vi "CameraTesting3.vi"() -> ()   [LabVIEW 2019]
doc: "The myRIO Project template acquires acceleration data from the onboard accelerometer and displays the changes of acceleration values in a waveform chart."
uses:
  <vilib>/myRIO/Express VI/Onboard IO/Encoder/Encoder Express VI.xnode
  <vilib>/myRIO/Common/Instrument Driver Framework/myRIO v1.0/Encoder/typedefs/Encoder Count Direction Enum.ctl
  <vilib>/myRIO/Instrument Drivers/Onboard IO/Encoder/typedefs/Encoder Reference.ctl
  <vilib>/myRIO/Instrument Drivers/Onboard IO/Encoder/Encoder.lvlib
  <vilib>/myRIO/Common/Instrument Driver Framework/myRIO v1.0/Encoder/typedefs/Encoder Channels Enum.ctl
  <vilib>/myRIO/Common/Instrument Driver Framework/Utilities/typedefs/myRIO Generic Hardware Reference.ctl
  <vilib>/myRIO/Common/Instrument Driver Framework/Utilities/typedefs/myRIO v1.0 Reference.ctl
  <vilib>/myRIO/Common/Instrument Driver Framework/Utilities/typedefs/Generic FPGA Reference.ctl
  <vilib>/myRIO/Common/Instrument Driver Framework/Utilities/typedefs/Hardware Version Enum.ctl
  <vilib>/myRIO/Common/Instrument Driver Framework/myRIO v1.0/Encoder/typedefs/Encoder Signal Mode.ctl
  <vilib>/myRIO/Instrument Drivers/Onboard IO/Encoder/vis/Read.vi
  <vilib>/myRIO/Instrument Drivers/Onboard IO/Encoder/vis/myRIO Encoder Open.xnode
  <vilib>/userdefined/High Color/nirio_resource_hc.ctl
  <vilib>/myRIO/Common/Instrument Driver Framework/myRIO v1.0/Encoder/typedefs/Encoder Configuration v1.0.ctl
  <vilib>/myRIO/Common/Instrument Driver Framework/myRIO v1.0/Encoder/vis/myRIO v1.1 Open Encoder.vi
  <vilib>/myRIO/Common/Instrument Driver Framework/myRIO v1.0/Encoder/vis/myRIO v1.0 Configure Encoder.vi
  <vilib>/myRIO/Common/Instrument Driver Framework/Utilities/vis/Is FPGA Ref Available.vi
  <vilib>/myRIO/Express VI/Onboard IO/DO/DO Express VI.xnode
  <vilib>/myRIO/Instrument Drivers/Onboard IO/DIO/typedefs/DIO Reference.ctl
  <vilib>/myRIO/Instrument Drivers/Onboard IO/DIO/DIO.lvlib
  <vilib>/myRIO/Common/Instrument Driver Framework/myRIO v1.0/DIO/typedefs/DIO Channels List.ctl
  <vilib>/myRIO/Common/Instrument Driver Framework/myRIO v1.0/DIO/typedefs/DIO Channels Enum.ctl
  <vilib>/myRIO/Instrument Drivers/Onboard IO/DIO/vis/Write.vi
  <vilib>/myRIO/Instrument Drivers/Onboard IO/DIO/vis/myRIO DIO Open.xnode
  <vilib>/myRIO/Common/Instrument Driver Framework/myRIO v1.0/DIO/vis/myRIO v1.1 Open DIO.vi
  <vilib>/Analysis/NI_AALBase.lvlib
panel:
  out "Pause":i32
  out "WaitTime":dbl=1000.0
  out "SquareWave":dbl
  out "FrameRate":i32=30
  out "Stop":bool
  out "VidTS":dbl[][](array[numeric])
  out "GoVid":i32=1
  out "VidFrameClock":i32
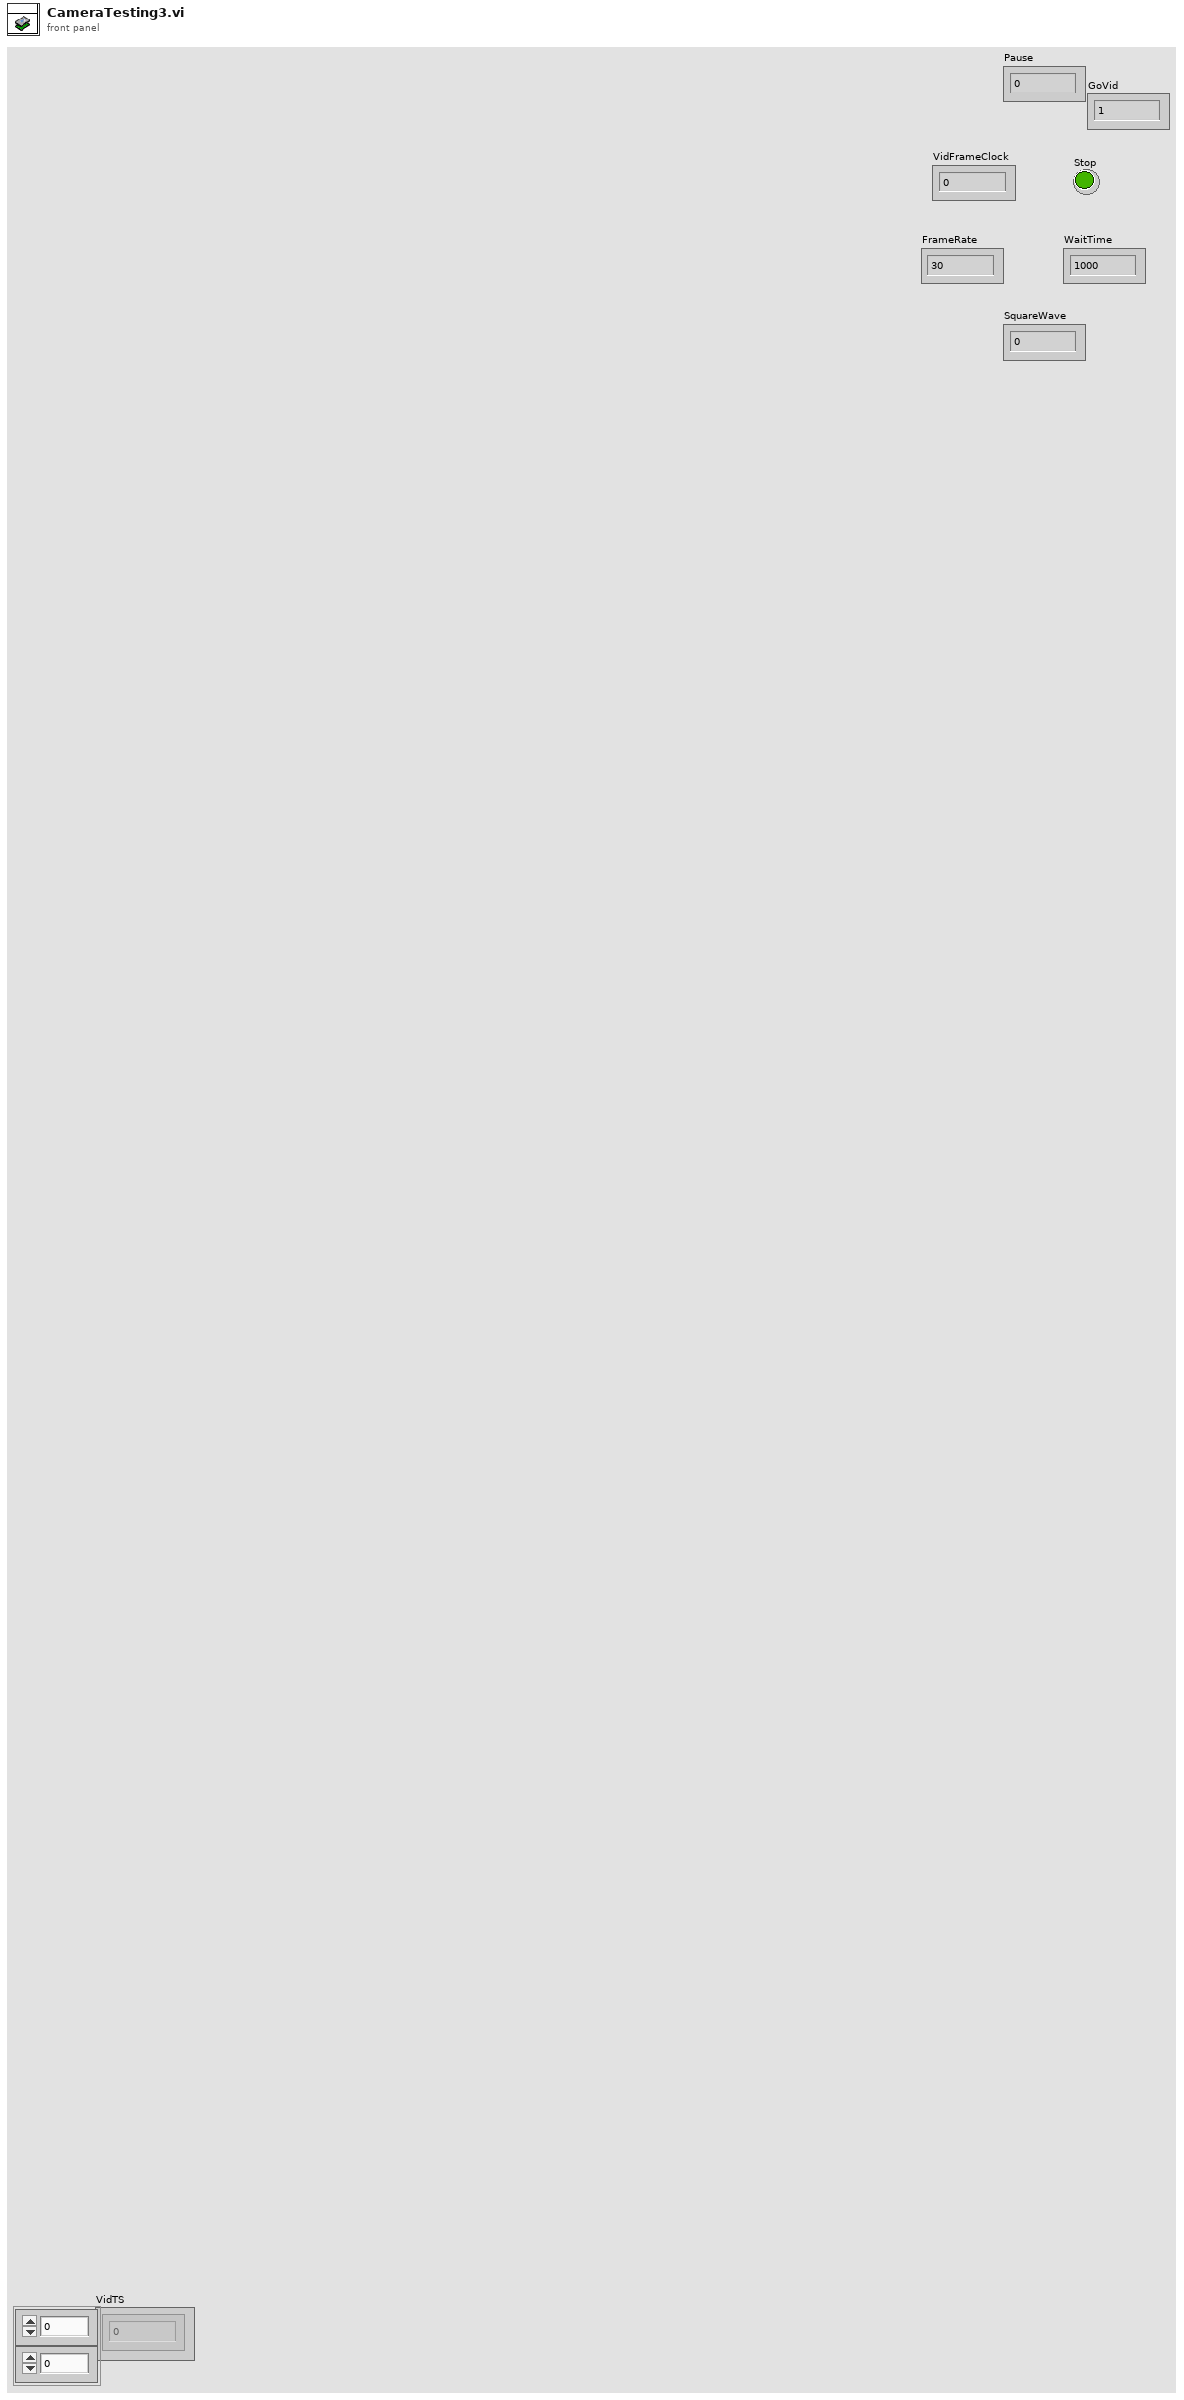
[diagram p1: front panel]
types:
  T1 = typedef "Encoder.lvlib/Encoder Reference.ctl" = cluster{"myRIO Reference":T2, "Encoder Channels Enum":T6}
  T2 = typedef "myRIO Generic Hardware Reference.ctl" = cluster{"myRIO Model":T3, "myRIO Hardware Reference":T4}
  T3 = typedef "Hardware Version Enum.ctl" = enum16{"Unknown", "myRIO-1900", "myRIO-1950", "roboRIO", "NI ELVIS RIO CM", "ELVIS III"}
  T4 = typedef "myRIO v1.0 Reference.ctl" = cluster{"Generic FPGA Reference":T5, "Allow multiple opens":bool}
  T5 = typedef "Generic FPGA Reference.ctl" = refnum<k20>
  T6 = typedef "Encoder Channels Enum.ctl" = enum16{"Not Connected", "C/ENC0", "C/ENC1", "A/ENC", "A/ENC0", "A/ENC1", "A/ENC2", "A/ENC3", "A/ENC4", "A/ENC5", "A/ENC6", "A/ENC7", "A/ENC8", "A/ENC9", "B/ENC", "B/ENC0", "B/ENC1", "B/ENC2", "B/ENC3", "B/ENC4", "B/ENC5", "B/ENC6", "B/ENC7", "B/ENC8", "B/ENC9", "DIO/ENC0", "DIO/ENC1", "DIO/ENC2", "DIO/ENC3", "DIO/ENC4"}
  T7 = typedef "Encoder Signal Mode.ctl" = enum16{"Quadrature phase signal", "Step and direction signal"}
  T8 = typedef "nirio_resource_hc.ctl" = tag
  T9 = typedef "NI_Matrix.lvlib/RealMatrix.ctl" = dbl[][]
  T10 = typedef "DIO.lvlib/DIO Reference.ctl" = cluster{"myRIO Reference":T2, "DIO Channels List":T11}
  T11 = typedef "DIO Channels List.ctl" = T12[]
  T12 = typedef "DIO Channels Enum.ctl" = enum16{"Not Connected", "C/DIO0", "C/DIO1", "C/DIO2", "C/DIO3", "C/DIO4", "C/DIO5", "C/DIO6", "C/DIO7", "A/DIO0", "A/DIO1", "A/DIO2", "A/DIO3", "A/DIO4", "A/DIO5", "A/DIO6", "A/DIO7", "A/DIO8", "A/DIO9", "A/DIO10", "A/DIO11", "A/DIO12", "A/DIO13", "A/DIO14", "A/DIO15", "A/DIO16", "A/DIO17", "A/DIO18", "A/DIO19", "B/DIO0", "B/DIO1", "B/DIO2", "B/DIO3", "B/DIO4", "B/DIO5", "B/DIO6", "B/DIO7", "B/DIO8", "B/DIO9", "B/DIO10", "B/DIO11", "B/DIO12", "B/DIO13", "B/DIO14", "B/DIO15", "B/DIO16", "B/DIO17", "B/DIO18", "B/DIO19", "LED0", "LED1", "LED2", "LED3", "Button0", "DIO/DIO0", "DIO/DIO1", "DIO/DIO2", "DIO/DIO3", "DIO/DIO4", "DIO/DIO5", "DIO/DIO6", "DIO/DIO7", "DIO/DIO8", "DIO/DIO9", "SPI/CS0", "SPI/CS1", "SPI/CS2", "SPI/CS3", "LED RADIO (Green)", "LED RADIO (Red)", "LED COMM (Green)", "LED COMM (Red)", "LED MODE (Green)", "LED MODE (Red)"}
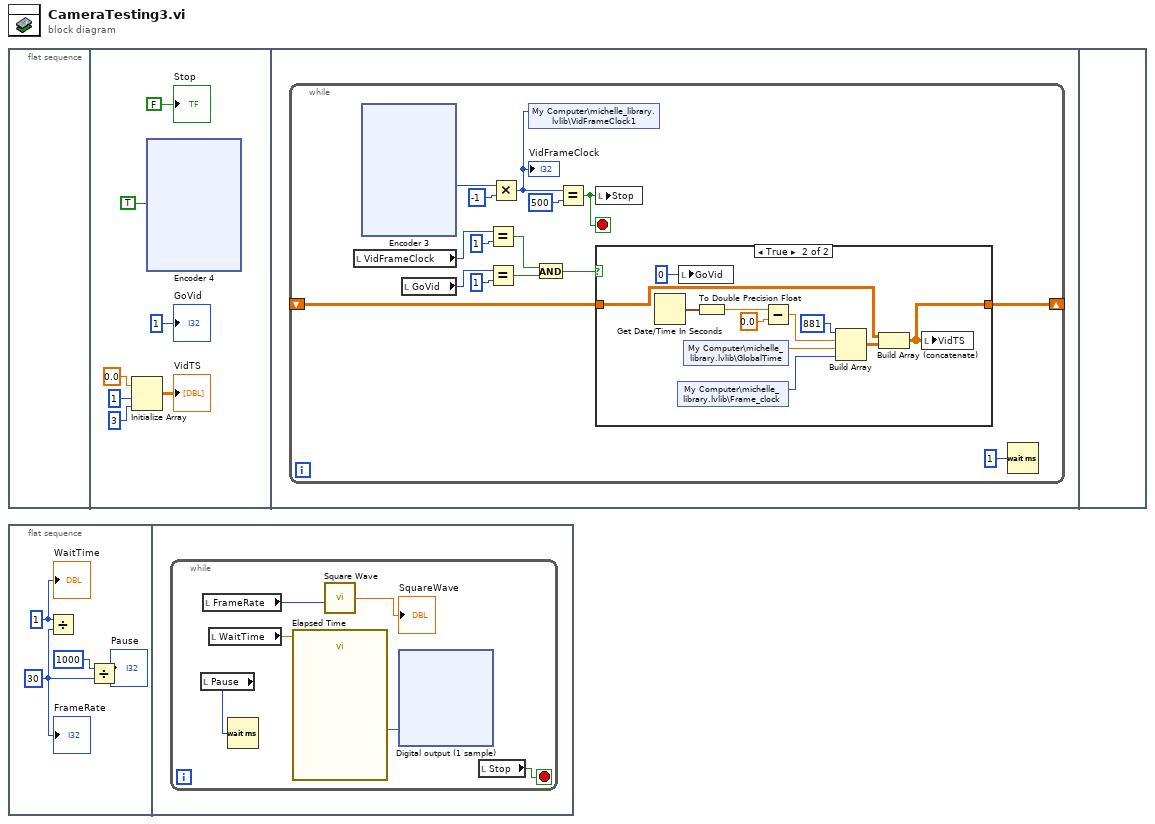
[diagram p0: block diagram]
diagram:
  n1 = flat-sequence {
    frame #0 {
    }
    frame #1 {
      n2 = Initialize Array(0.0, 1, 3) -> (→"VidTS":dbl[][])
      n3 = xnode "Encoder 4"("Reset Counter"=TRUE) -> ()  [unwired: 1 in, 4 out]
      "GoVid" <- 1
      "Stop" <- FALSE
    }
    frame #2 {
      n4 = while {
        shift-right: [w60] -> _
        shift-left: _ -> [w61]
        stop <- w65 stop-if-true
        n5 = local read "VidFrameClock"() -> (w59:i32)
        n6 = xnode "Encoder 3"() -> ("Counter Value"=w67:i32)  [unwired: 2 in, 3 out]
        n7 = local read "GoVid"() -> (w55:i32)
        n8 = Equal?(x=w59, y=1) -> (x = y?=w58:bool)
        n9 = Equal?(x=w55, y=1) -> (x = y?=w54:bool)
        n10 = Multiply(x=w67, y=-1) -> (x*y=w64:i32)
        "VidFrameClock" <- w64
        n11 = shared-variable "My Computer\\michelle_library.lvlib\\VidFrameClock1"(w64) -> ()  [unwired: 1 in, 1 out]
        n12 = And(x=w58, y=w54) -> (x .and. y?=w57:bool)
        n13 = Equal?(x=w64, y=500) -> (x = y?=w65:bool)
        n14 = local write "Stop"(w65) -> ()
        n15 = case shown="True" w57 {
          tunnel: w61 -> [w69 w73]
          tunnel: [w69 w72] -> w60
          frame False {
          }
          frame True {
            n16 = Get Date/Time In Seconds() -> (seconds since 1Jan1904=w80:timestamp)
            n17 = shared-variable "My Computer\\michelle_library.lvlib\\Frame_clock"() -> (w77:u32)  [unwired: 1 in, 1 out]
            n18 = local write "GoVid"(0) -> ()
            n19 = shared-variable "My Computer\\michelle_library.lvlib\\GlobalTime"() -> (w76:dbl)  [unwired: 1 in, 1 out]
            n20 = To Double Precision Float(number=w80) -> (double precision float=w79:dbl)
            n21 = Subtract(x=w79, y=0.0) -> (x-y=w78:dbl)
            n22 = Build Array(881, w78, w76, w77) -> (w75:T9)
            n23 = Build Array (concatenate) ("Build Matrix")(w73, w75) -> (w72:T9)
            n24 = local write "VidTS"(w72) -> ()
          }
        }
        n25 = Wait (ms)(milliseconds to wait=u32 1) -> ()  [unwired: 1 out]
      }
    }
    frame #3 {
    }
  }
  n26 = flat-sequence {
    frame #0 {
      w129 = 1
      w127 = 30
      n27 = Divide(x=w129, y=w127) -> ()  [unwired: 1 out]
      n28 = Divide(x=1000, y=w127) -> ()  [unwired: 1 out]
      "FrameRate" <- w127
      "WaitTime" <- w129
    }
    frame #1 {
      n29 = while {
        stop <- w135 stop-if-true
        n30 = local read "Pause"() -> (w130:i32)
        n31 = local read "FrameRate"() -> (w133:i32)
        n32 = local read "WaitTime"() -> (w132:dbl)
        n33 = Wait (ms)(milliseconds to wait=w130) -> ()  [unwired: 1 out]
        n34 = call "Elapsed Time"("Time Target (s)"=w132) -> ("Time has Elapsed"=w131:bool)  [unwired: 11 in, 7 out]
        n35 = call <vilib>:"Square Wave.vi"("frequency"=w133) -> ("phase out"=→"SquareWave":dbl)  [unwired: 5 in, 2 out]
        n36 = xnode "Digital output (1 sample)"("VidTrig (B/DIO5 (Pin 21))"=w131) -> ()  [unwired: 1 in, 1 out]
        n37 = local read "Stop"() -> (w135:bool)
      }
    }
  }
